vi "Limelight Create File to Record Values.vi"() -> ()   [LabVIEW 2020]
uses:
  Framework/Robot Global Data.vi
panel:
  out "error out":errorcluster
  out "Limelight Values Filepath":path
  out "Deleted Previous Limelight File":path
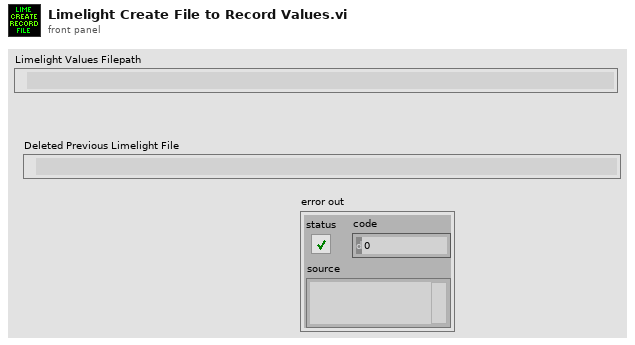
[diagram p1: front panel]
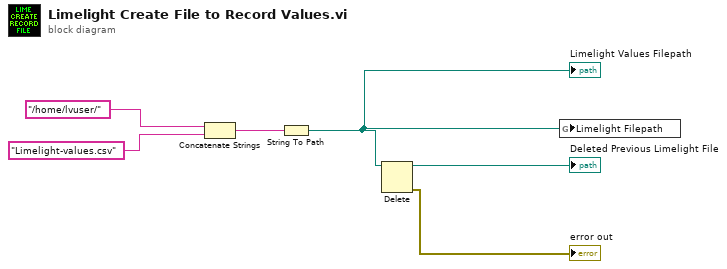
[diagram p0: block diagram]
diagram:
  n1 = Concatenate Strings("/home/lvuser/", "Limelight-values.csv") -> (w3:string)
  n2 = String To Path(string=w3) -> (path=w4:path)
  "Limelight Values Filepath" <- w4
  n3 = Delete(path (use dialog)=w4) -> (deleted path=→"Deleted Previous Limelight File":path, error out=→"error out":errorcluster)  [unwired: 4 in, 1 out]
  n4 = global write "Robot Global Data.vi" "Limelight Filepath"(w4) -> ()
